vi "VisionGlb.vi"() -> ()   [LabVIEW 2019]
panel:
  out "Root Path":path
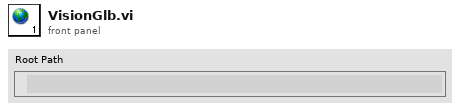
[diagram p1: front panel]
diagram:
